vi "Execute.vi"(8 "error in (no error)":errorcluster, 10 "Execution in":refnum<data-value>, 11 "CallEXEStepBase in":refnum<class "CallEXEStep.lvclass">) -> (0 "error out":errorcluster, 1 "Output Values":cluster{"Name":string, "Variant Data":variant}[](array[cluster]), 3 "CallEXEStepBase out":refnum<class "CallEXEStep.lvclass">)   [LabVIEW 2015, in "CallEXEStep.lvclass"]
uses:
  CallEXEStep.lvclass
  Execution.lvclass
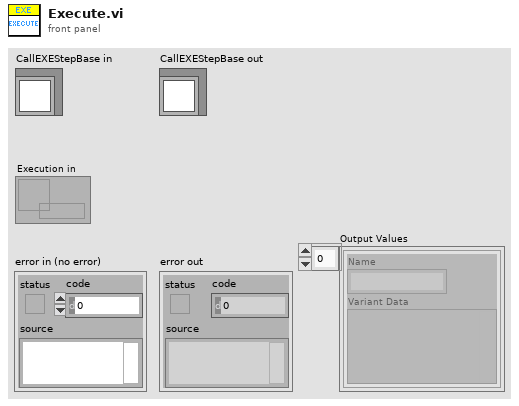
[diagram p1: front panel]
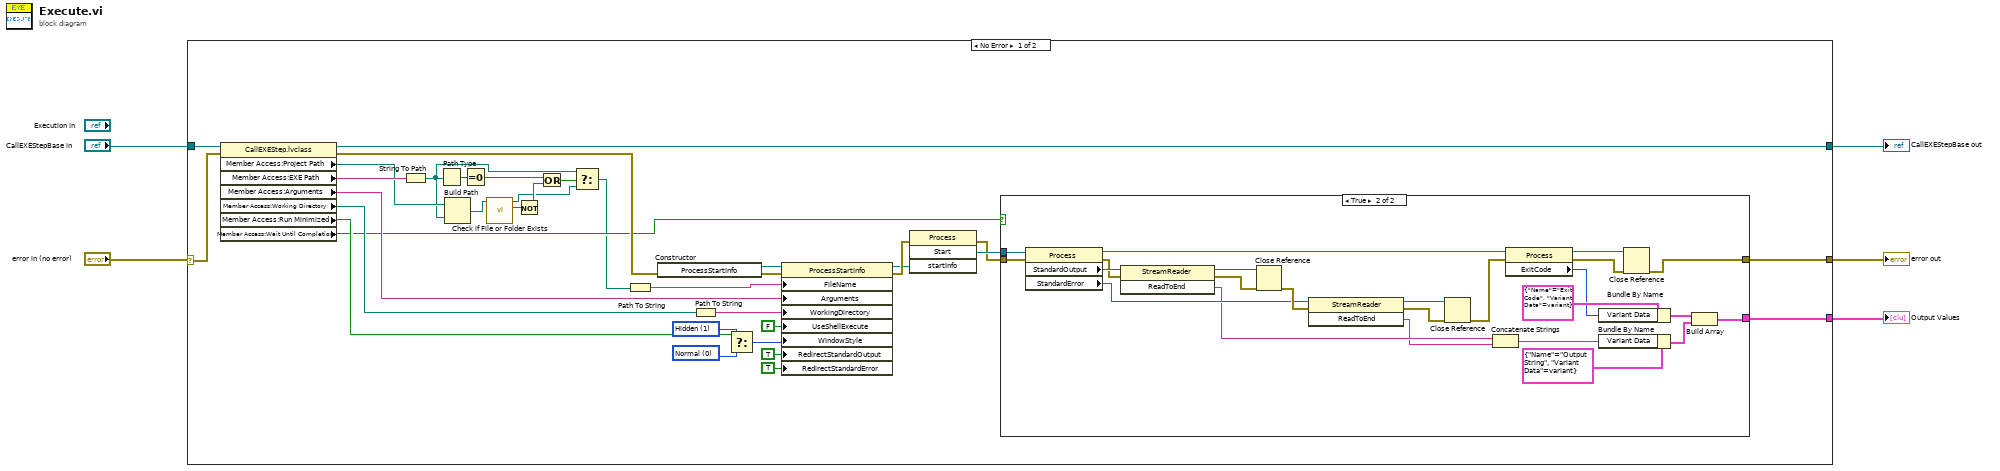
[diagram p0: block diagram]
diagram:
  n1 = case shown="No Error" "error in (no error)" {
    selector: "error in (no error)" -> [w24 w67]
    tunnel: "CallEXEStepBase in" -> [w40 w66]
    tunnel: [w13 w67] -> w3
    tunnel: [w39 w66] -> w2
    tunnel: [w12 _] -> w1
    frame No Error {
      w29 = 1 items=["Normal", "Hidden", "Minimized", "Maximized"] ("WindowStyle")
      w30 = 0 items=["Normal", "Hidden", "Minimized", "Maximized"] ("WindowStyle")
      n2 = property class="CallEXEStep.lvclass"(reference=w40, error in=w24) -> (reference out=w39:refnum<class "CallEXEStep.lvclass">, error out=w23:errorcluster, "Member Access:Project Path"=w18:path, "Member Access:EXE Path"=w20:string, "Member Access:Arguments"=w34:string, "Member Access:Working Directory"=w33:path, "Member Access:Run Minimized"=w27:bool, "Member Access:Wait Until Completion"=w22:bool)
      n3 = String To Path(string=w20) -> (path=w17:path)
      n4 = Path Type(1:w17) -> (0:w19:i16)
      n5 = Build Path(base path=w18, name or relative path=w17) -> (appended path=w11:path)
      n6 = Equal To 0?(x=w19) -> (x = 0?=w8:bool)
      n7 = call <vilib>:"Check if File or Folder Exists.vi"("path"=w11) -> ("file or folder exists?"=w10:bool, "dup path"=w6:path)  [unwired: 8 in, 1 out]
      n8 = Not(x=w10) -> (.not. x?=w9:bool)
      n9 = Or(x=w8, y=w9) -> (x .or. y?=w7:bool)
      n10 = Select(t=w17, s=w7, f=w6) -> (s? t:f=w16:path)
      n11 = Path To String(path=w16) -> (string=w15:string)
      n12 = constructor class="ProcessStartInfo"(error in=w23) -> (reference out=w35:refnum<k24>, error out=w36:errorcluster)  [unwired: 2 in, 1 out]
      n13 = Path To String(path=w33) -> (string=w32:string)
      n14 = Select(t=w29, s=w27, f=w30) -> (s? t:f=w28:i32)
      n15 = property class="ProcessStartInfo"(reference=w35, error in=w36, "FileName"=w15, "Arguments"=w34, "WorkingDirectory"=w32, "UseShellExecute"=FALSE, "WindowStyle"=w28, "RedirectStandardOutput"=TRUE, "RedirectStandardError"=TRUE) -> (reference out=w37:refnum<k24>, error out=w38:errorcluster)
      n16 = invoke class="Process" method="Start"(error in=w38, "startInfo"=w37) -> (error out=w25:errorcluster, "Start"=w26:refnum<k24>)  [unwired: 2 in, 2 out]
      n17 = case shown="True" w22 {
        tunnel: w26 -> [_ w60]
        tunnel: w25 -> [w41 w59]
        tunnel: [w41 w61] -> w13
        tunnel: [_ w42] -> w12
        frame False {
        }
        frame True {
          n18 = property class="Process"(reference=w60, error in=w59) -> (reference out=w58:refnum<k24>, error out=w64:errorcluster, "StandardOutput"=w65:refnum<k24>, "StandardError"=w52:refnum<k24>)
          n19 = invoke class="StreamReader" method="ReadToEnd"(reference=w65, error in=w64) -> (reference out=w63:refnum<k24>, error out=w62:errorcluster, "ReadToEnd"=w51:string)  [unwired: 1 in]
          n20 = Close Reference(reference=w63, error in (no error)=w62) -> (error out=w53:errorcluster)
          n21 = invoke class="StreamReader" method="ReadToEnd"(reference=w52, error in=w53) -> (reference out=w54:refnum<k24>, error out=w55:errorcluster, "ReadToEnd"=w50:string)  [unwired: 1 in]
          n22 = Close Reference(reference=w54, error in (no error)=w55) -> (error out=w49:errorcluster)
          n23 = Concatenate Strings(w51, w50) -> (w45:string)
          n24 = property class="Process"(reference=w58, error in=w49) -> (reference out=w57:refnum<k24>, error out=w56:errorcluster, "ExitCode"=w47:i32)
          n25 = Bundle By Name(cluster=cluster{"Name":string, "Variant Data":variant} {"Name"="Exit Code", "Variant Data"=variant}, "Variant Data"=w47) -> (w44:cluster{"Name":string, "Variant Data":variant})
          n26 = Bundle By Name(cluster=cluster{"Name":string, "Variant Data":variant} {"Name"="Output String", "Variant Data"=variant}, "Variant Data"=w45) -> (w43:cluster{"Name":string, "Variant Data":variant})
          n27 = Close Reference(reference=w57, error in (no error)=w56) -> (error out=w61:errorcluster)
          n28 = Build Array(w44, w43) -> (w42:cluster{"Name":string, "Variant Data":variant}[])
        }
      }
    }
    frame Error {
    }
  }
  "error out" <- w3
  "CallEXEStepBase out" <- w2
  "Output Values" <- w1
